vi "Take Step.vi"(8 "error in (no error)":errorcluster, 10 "Mouse In":refnum<class "Mouse.lvclass">, 11 "Maze in":refnum<class "Maze.lvclass">) -> (0 "error out":errorcluster, 1 "Crash?":bool, 2 "Mouse":refnum<class "Mouse.lvclass">, 3 "Maze":refnum<class "Maze.lvclass">, 4 "New Position":T1, 5 "Direction":T2, 6 "Old Position":T1)   [LabVIEW 2020, in "Maze.lvlib" / "Maze.lvclass"]
doc: "This is the VI meant to be called by the App to progress the exploration by 1 step. It calls into the community scoped Take Step in the mouse class which then manages the mouse state."
uses:
  Maze.lvclass
  Mouse/Mouse.lvclass
  Position.ctl
  Direction.ctl
  Maze.lvlib
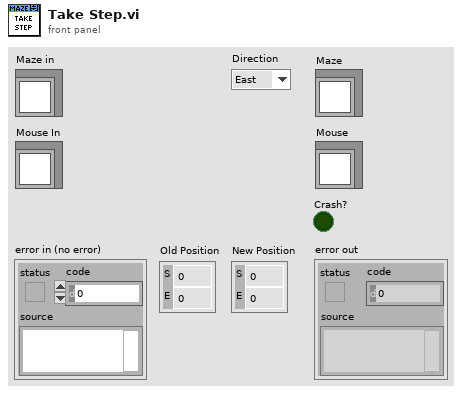
[diagram p1: front panel]
types:
  T1 = typedef "Maze.lvlib/Position.ctl" = cluster{"S":i32, "E":i32}
  T2 = typedef "Maze.lvlib/Direction.ctl" = enum8{"East", "North", "West", "South"}
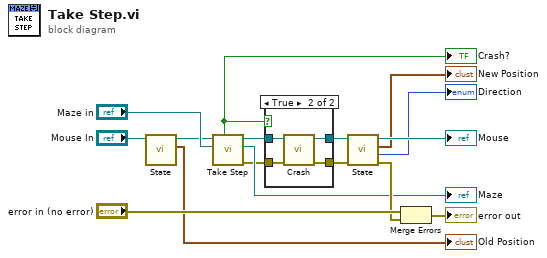
[diagram p0: block diagram]
diagram:
  n1 = call "State.vi"("Mouse in"="Mouse In") -> ("Position"=→"Old Position":T1, "Mouse out"=w8:refnum<class "Mouse.lvclass">)  [unwired: 7 in, 2 out]
  n2 = call "Take Step.vi"("Maze In"="Maze in", "Mouse in"=w8) -> ("error out"=w3:errorcluster, "Maze"=→"Maze":refnum<class "Maze.lvclass">, "Mouse out"=w5:refnum<class "Mouse.lvclass">, "Crash?"=w6:bool)  [unwired: 5 in, 1 out]
  "Crash?" <- w6
  n3 = case shown="True" w6 {
    tunnel: w5 -> [w18 w22]
    tunnel: w3 -> [w17 w21]
    tunnel: [w17 w20] -> w2
    tunnel: [w18 w19] -> w1
    frame False {
    }
    frame True {
      n4 = call-dynamic "Crash.vi"("error in (no error)"=w21, "Mouse in"=w22) -> ("error out"=w20:errorcluster, "Mouse out"=w19:refnum<class "Mouse.lvclass">)  [unwired: 8 in]
    }
  }
  n5 = call "State.vi"("error in (no error)"=w2, "Mouse in"=w1) -> ("error out"=w10:errorcluster, "Direction"=→"Direction":T2, "Position"=→"New Position":T1, "Mouse out"=→"Mouse":refnum<class "Mouse.lvclass">)  [unwired: 6 in]
  n6 = Merge Errors("error in (no error)", w10) -> (→"error out":errorcluster)
